vi "ReachGoal.vi"(8 "error in":errorcluster, 10 "Goal point":T4) -> (0 "error out":errorcluster)   [LabVIEW 2009, in "Main.lvlib"]
doc: "Main subroutine for reach specified point."
uses:
  Main.lvlib
  Drive/Drive_Point.ctl
  MainVariables.lvlib
  NetworkVarTarget.lvlib
  Drive/Drive_Utils.lvlib
  Drive.lvlib
panel:
  out "Objects bottom cords":T1(array[cluster])
  out "Walls":T2(array[cluster])
  out "state out":T3
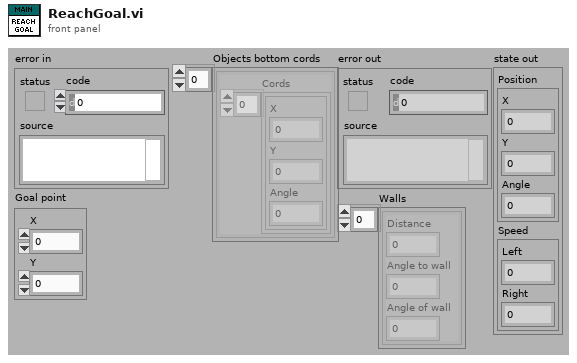
[diagram p1: front panel]
types:
  T1 = cluster{"Cords":cluster{"X":dbl, "Y":dbl, "Angle":dbl}[]}[]
  T2 = cluster{"Distance":dbl, "Angle to wall":dbl, "Angle of wall":dbl}[]
  T3 = cluster{"Position":cluster{"X":dbl, "Y":dbl, "Angle":dbl}, "Speed":cluster{"Left":dbl, "Right":dbl}}
  T4 = typedef "Drive.lvlib/Drive_Point.ctl" = cluster{"X":dbl, "Y":dbl}
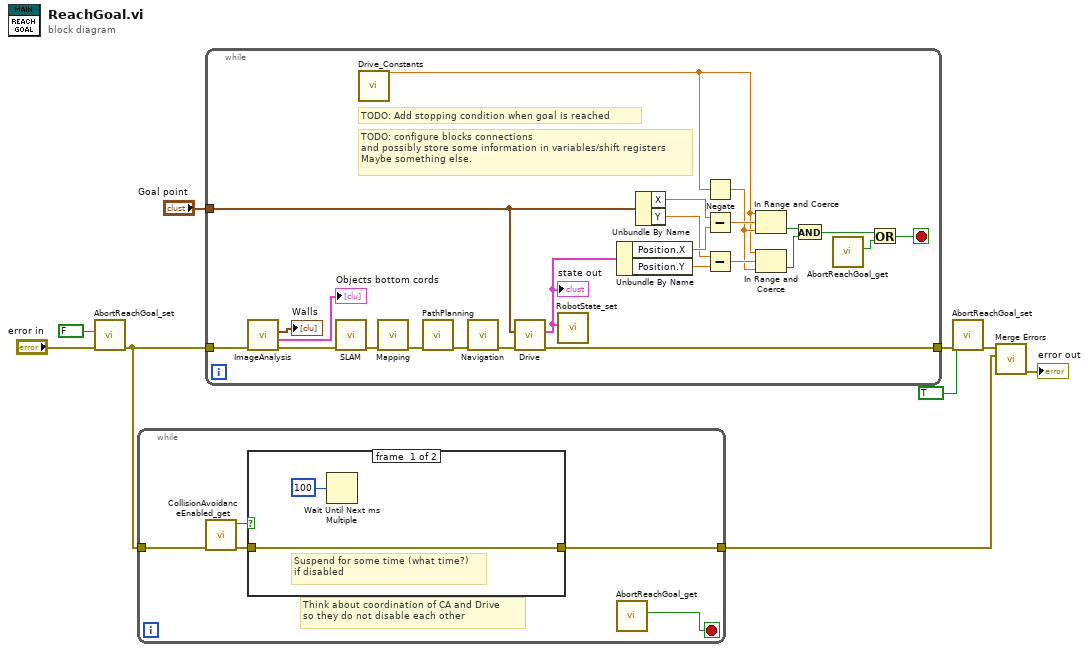
[diagram p0: block diagram]
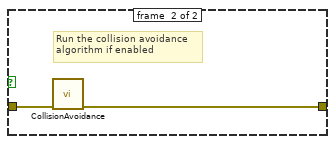
[diagram p2: hidden frame]
diagram:
  n1 = call "AbortReachGoal_set.vi"("error in (no error)"="error in", "Abort? (F)"=FALSE) -> ("error out"=w5:errorcluster)  [unwired: 9 in]
  n2 = while {
    tunnel: [w12] -> w9
    tunnel: w5 -> [w11]
    stop <- w10 stop-if-true
    # "Think about coordination of CA and Drive\nso they do not disable each other"
    n3 = call "CollisionAvoidanceEnabled_get.vi"("error in (no error)"=w11) -> ("error out"=w13:errorcluster, "Enabled"=w14:bool)  [unwired: 9 in]
    n4 = case shown="True" w14 {
      tunnel: w13 -> [w15 w18]
      tunnel: [w15 w17] -> w12
      frame #0 {
        # "Suspend for some time (what time?)\nif disabled"
        n5 = Wait Until Next ms Multiple(millisecond multiple=u32 100) -> ()  [unwired: 1 out]
      }
      frame #1 {
        # "Run the collision avoidance\nalgorithm if enabled"
        n6 = call "CollisionAvoidance.vi"("error in"=w18) -> ("error out"=w17:errorcluster)  [unwired: 10 in]
      }
    }
    n7 = call "AbortReachGoal_get.vi"() -> ("Abort"=w10:bool)  [unwired: 10 in, 1 out]
  }
  n8 = while {
    tunnel: w5 -> [w42]
    tunnel: [w38] -> w2
    tunnel: "Goal point" -> [w30]
    stop <- w32 stop-if-true
    # "TODO: Add stopping condition when goal is reached"
    # "TODO: configure blocks connections\nand possibly store some information in variables/shift registers\nMaybe something else."
    n9 = call "ImageAnalysis.vi"("error in"=w42) -> ("error out"=w41:errorcluster, "Objects bottom cords"=→"Objects bottom cords":T1, "Walls"=→"Walls":T2)  [unwired: 8 in]
    n10 = call "SLAM.vi"("error in"=w41) -> ("error out"=w40:errorcluster)  [unwired: 10 in]
    n11 = call "Drive_Constants.vi"() -> ("Position accuracy (m)"=w19:dbl)  [unwired: 22 in, 5 out]
    n12 = call "Mapping.vi"("error in"=w40) -> ("error out"=w36:errorcluster)  [unwired: 10 in]
    n13 = call "PathPlanning.vi"("error in"=w36) -> ("error out"=w37:errorcluster)  [unwired: 10 in]
    n14 = call "Navigation.vi"("error in"=w37) -> ("error out"=w39:errorcluster)  [unwired: 9 in, 1 out]
    n15 = call "Drive.vi"("error in"=w39, "Relative Coordinates"=w30) -> ("error out"=w38:errorcluster, "state out"=w31:T3)  [unwired: 8 in]
    "state out" <- w31
    n16 = call "RobotState_set.vi"("RobotState"=w31) -> ()  [unwired: 10 in, 1 out]
    n17 = Unbundle By Name(w31) -> ("Position.X"=w24:dbl, "Position.Y"=w22:dbl)
    n18 = Unbundle By Name(w30) -> ("X"=w25:dbl, "Y"=w23:dbl)
    n19 = Negate(x=w19) -> (-x=w20:dbl)
    n20 = Subtract(x=w25, y=w24) -> (x-y=w26:dbl)
    n21 = Subtract(x=w23, y=w22) -> (x-y=w21:dbl)
    n22 = In Range and Coerce(upper limit=w19, x=w26, lower limit=w20) -> (In Range?=w29:bool)  [unwired: 1 out]
    n23 = In Range and Coerce(upper limit=w19, x=w21, lower limit=w20) -> (In Range?=w28:bool)  [unwired: 1 out]
    n24 = And(x=w29, y=w28) -> (x .and. y?=w27:bool)
    n25 = call "AbortReachGoal_get.vi"() -> ("Abort"=w33:bool)  [unwired: 10 in, 1 out]
    n26 = Or(x=w27, y=w33) -> (x .or. y?=w32:bool)
  }
  n27 = call "AbortReachGoal_set.vi"("error in (no error)"=w2, "Abort? (F)"=TRUE) -> ("error out"=w3:errorcluster)  [unwired: 9 in]
  n28 = call <vilib>:"Merge Errors.vi"("error in 2 (no error)"=w9, "error in 1 (no error)"=w3) -> ("error out"=→"error out":errorcluster)  [unwired: 5 in]
